vi "Top Level.vi"() -> ()   [LabVIEW 2017]
uses:
  Modules/Events/Events.lvlib
  Modules/Monochromator/Monochromator.lvlib
  Modules/Shutter Module/Shutter.lvlib
  Modules/UI/UI.lvlib
  Modules/DAQ/DAQ.lvlib
  Modules/Scope/Scope.lvlib
  Modules/File IO/File IO.lvlib
  Modules/Colour Wheel/Colour Wheel.lvlib
  Modules/Processing/Processing.lvlib
  Modules/System Control/Main controller.lvlib
panel:
  in  "Simulate hardware?":bool
  # "Optical Software"
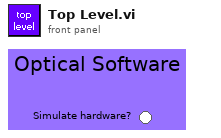
[diagram p1: front panel]
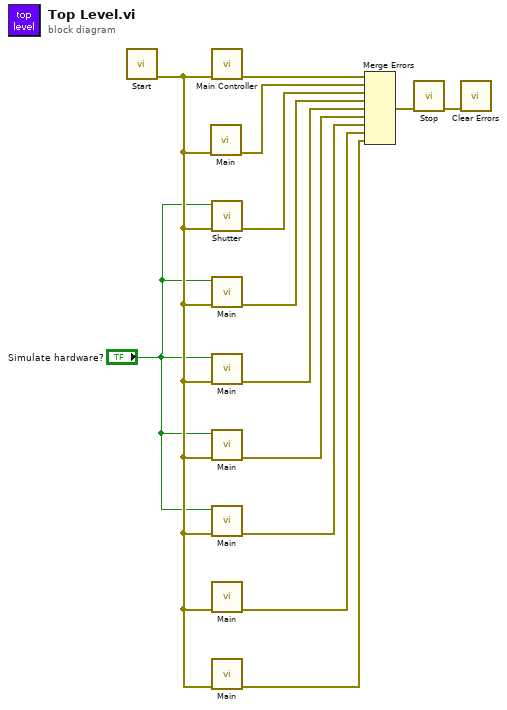
[diagram p0: block diagram]
diagram:
  n1 = call "Start.vi"() -> ("Error Out"=w3:errorcluster)  [unwired: 11 in]
  n2 = call "Main.vi"("Error In"=w3) -> ("Error Out"=w10:errorcluster)  [unwired: 10 in]
  n3 = call "Main Controller.vi"("Error In"=w3) -> ("Error Out"=w2:errorcluster)  [unwired: 10 in]
  n4 = call "Shutter.vi"("Error In"=w3, "Simulate hardware?"="Simulate hardware?") -> ("Error Out"=w12:errorcluster)  [unwired: 9 in]
  n5 = call "Main.vi"("Error In"=w3, "Simulate hardware?"="Simulate hardware?") -> ("Error Out"=w11:errorcluster)  [unwired: 9 in]
  n6 = call "Main.vi"("Error In"=w3, "Simulate hardware?"="Simulate hardware?") -> ("Error Out"=w5:errorcluster)  [unwired: 9 in]
  n7 = call "Main.vi"("Error In"=w3, "Simulate hardware?"="Simulate hardware?") -> ("Error Out"=w9:errorcluster)  [unwired: 9 in]
  n8 = call "Main.vi"("Error In"=w3, "Simulate hardware?"="Simulate hardware?") -> ("Error Out"=w8:errorcluster)  [unwired: 9 in]
  n9 = call "Main.vi"("Error In"=w3) -> ("Error Out"=w7:errorcluster)  [unwired: 10 in]
  n10 = call "Main.vi"("Error In"=w3) -> ("Error Out"=w4:errorcluster)  [unwired: 10 in]
  n11 = Merge Errors(w2, w10, w12, w11, w5, w9, w8, w7, w4) -> (w13:errorcluster)
  n12 = call "Stop.vi"("Error In"=w13) -> ("Error Out"=w6:errorcluster)  [unwired: 10 in]
  n13 = call <vilib>:"Clear Errors.vi"("error in (no error)"=w6) -> ()  [unwired: 5 in, 2 out]
